vi "JOG模式.vi"() -> ()   [LabVIEW 2023]
uses:
  <vilib>/Instr/_visa.llb/VISA Configure Serial Port (Instr).vi
panel:
  in  "stop bits (10: 1 bit)":u16(ring)=10 caption="停止位（10: 1位）" items=["1.0"=10, "1.5"=15, "2.0"=20]
  in  "parity (0:none)":enum16{"None", "Odd", "Even", "Mark", "Space"}(ring) caption="奇偶（0:无）"
  in  "data bits (8)":u16=8 caption="数据比特(8)" min=5 max=8 step=1
  in  "baud rate (9600)":u32=9600 caption="波特率(9600)"
  in  "VISA resource name":refnum<visa-resource-name> caption="VISA资源名称"
  out "错误输出":errorcluster
  out "返回数 2":u32
  out "读取缓冲区":string
  out "返回数":u32
  out "Write String":string
  in  "-5":bool
  in  "停止":bool
  in  "+5":bool
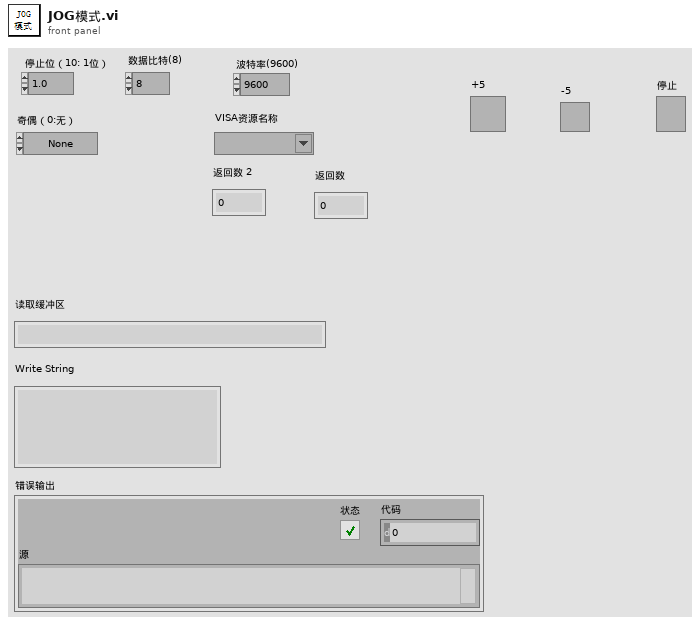
[diagram p1: front panel]
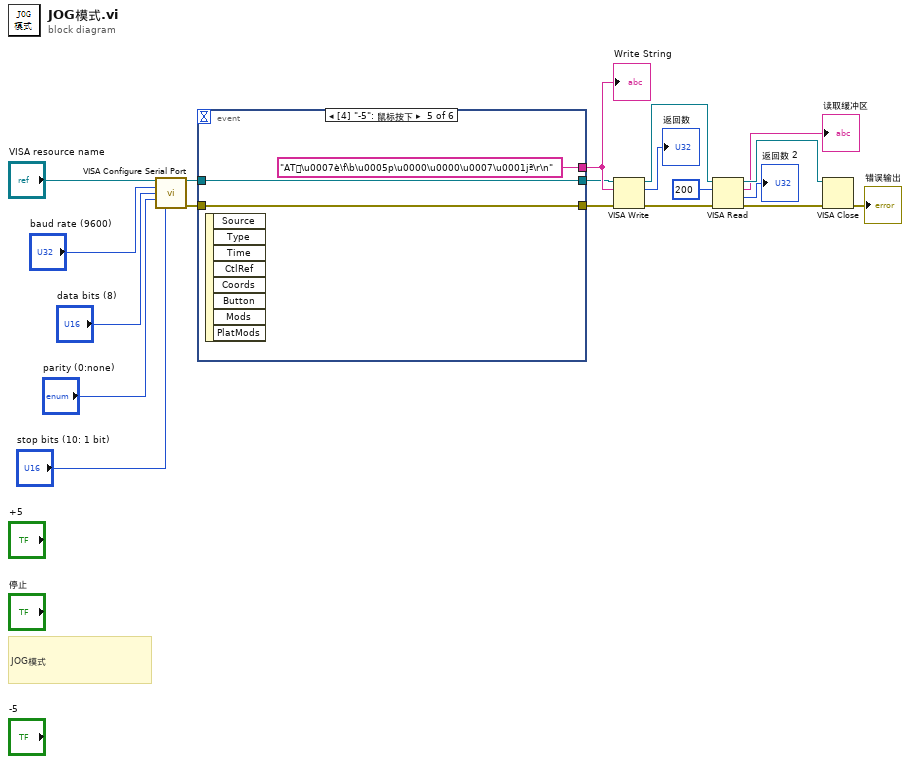
[diagram p0: block diagram]
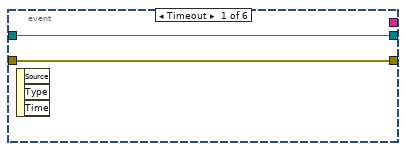
[diagram p2: hidden frame]
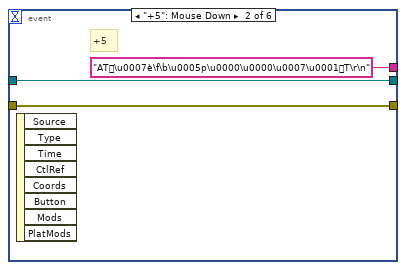
[diagram p3: hidden frame]
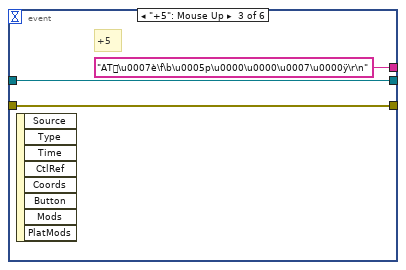
[diagram p4: hidden frame]
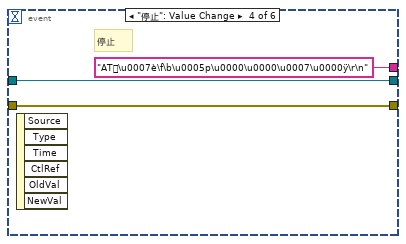
[diagram p5: hidden frame]
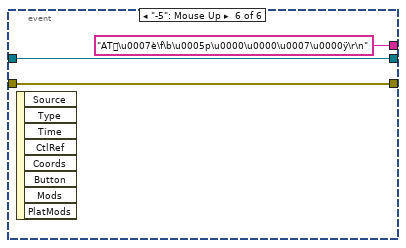
[diagram p6: hidden frame]
diagram:
  # "JOG模式"
  n1 = call-poly "VISA Configure Serial Port"("VISA resource name"="VISA resource name", "baud rate (9600)"="baud rate (9600)", "data bits (8)"="data bits (8)", "parity (0:none)"="parity (0:none)", "stop bits (10: 1 bit)"="stop bits (10: 1 bit)") -> ("VISA resource name out"=w4:refnum<visa-resource-name>, "error out"=w2:errorcluster)  [unwired: 9 in]
  n2 = event shown="[4] \"-5\": 鼠标按下" {
    selector: _ -> [_ _ _ _ _ _]
    dyn-events: _ -> [_ _ _ _ _ _]
    timeout: _ -> [_ _ _ _ _ _]
    tunnel: [_ "AT\u0007è\f\b\u0005p\u0000\u0000\u0007\u0001T\r\n" ("Write String") "AT\u0007è\f\b\u0005p\u0000\u0000\u0007\u0000ÿ\r\n" ("Write String") "AT\u0007è\f\b\u0005p\u0000\u0000\u0007\u0000ÿ\r\n" ("Write String") "AT\u0007è\f\b\u0005p\u0000\u0000\u0007\u0001jª\r\n" "AT\u0007è\f\b\u0005p\u0000\u0000\u0007\u0000ÿ\r\n"] -> w17
    tunnel: w4 -> [w21 w23 w25 w29 w32 w35]
    tunnel: [w21 w23 w25 w29 w32 w35] -> w3
    tunnel: w2 -> [w20 w22 w26 w28 w31 w34]
    tunnel: [w20 w22 w26 w28 w31 w34] -> w1
    event Timeout {
      n3 = event-data() -> ()  [unwired: 1 in, 3 out]
    }
    event "+5": Mouse Down {
      # "+5"
      n4 = event-data() -> ()  [unwired: 1 in, 8 out]
    }
    event "+5": Mouse Up {
      # "+5"
      n5 = event-data() -> ()  [unwired: 1 in, 8 out]
    }
    event "停止": Value Change {
      # "停止"
      n6 = event-data() -> ()  [unwired: 1 in, 6 out]
    }
    event "-5": Mouse Down {
      n7 = event-data() -> ()  [unwired: 1 in, 8 out]
    }
    event "-5": Mouse Up {
      n8 = event-data() -> ()  [unwired: 1 in, 8 out]
    }
  }
  "Write String" <- w17
  n9 = VISA Write(VISA resource name=w3, write buffer=w17, error in (no error)=w1) -> (VISA resource name out=w19:refnum<visa-resource-name>, return count=→"返回数":u32, error out=w18:errorcluster)
  n10 = VISA Read(VISA resource name=w19, byte count=u32 200 ("字节总数"), error in (no error)=w18) -> (VISA resource name out=w15:refnum<visa-resource-name>, read buffer=→"读取缓冲区":string, return count=→"返回数 2":u32, error out=w14:errorcluster)
  n11 = VISA Close(VISA resource name=w15, error in (no error)=w14) -> (error out=→"错误输出":errorcluster)
